vi "golpi_mpc_load_packages.vi"(8 "error in":errorcluster, 11 "golpi session":T1={"GOLPI ref"={"pipe handle"={"lv_proc.dll file path"=path "", "process instance handle"=[], "debug mode"=FALSE, "debug data"=[]}, "fast read timeout [ms]"=500, "fast read settle time [ms]"=10, "fast read to multiple [ms]"=1, "max elements per input line"=100, "slow read timeout [ms]"=5000, "stdin double format specifier"="%_16e", "max elements per stdout output column"=100, "console mode bitstream"=FALSE, "bitstream first read timeout [ms]"=1000, "bitstream read timeout [ms]"=50, "struct transfer possible"=FALSE, "matlab mode"=FALSE}, "idn str"="", "octave path"=path "C:/Octave364/Octave3.6.4_gcc4.6.2/bin", "work path"=path "C:/Octave364/Octave3.6.4_gcc4.6.2/bin", "start timeout [ms]"=15000, "clr cache"=FALSE, "console"=FALSE, "binary"=FALSE, "semaphore"=refnum, "initial command"="", "exit command"="", "matlab"=FALSE, "pkg list"=[]}) -> (0 "error out":errorcluster, 3 "golpi out":T1={"GOLPI ref"={"pipe handle"={"lv_proc.dll file path"=path "", "process instance handle"=[], "debug mode"=FALSE, "debug data"=[]}, "fast read timeout [ms]"=500, "fast read settle time [ms]"=10, "fast read to multiple [ms]"=1, "max elements per input line"=100, "slow read timeout [ms]"=5000, "stdin double format specifier"="%_16e", "max elements per stdout output column"=100, "console mode bitstream"=FALSE, "bitstream first read timeout [ms]"=1000, "bitstream read timeout [ms]"=50, "struct transfer possible"=FALSE, "matlab mode"=FALSE}, "idn str"="", "octave path"=path "C:/Octave364/Octave3.6.4_gcc4.6.2/bin", "work path"=path "C:/Octave364/Octave3.6.4_gcc4.6.2/bin", "start timeout [ms]"=15000, "clr cache"=FALSE, "console"=FALSE, "binary"=FALSE, "semaphore"=refnum, "initial command"="", "exit command"="", "matlab"=FALSE, "pkg list"=[]})   [LabVIEW 2020, in "GOLPI Multi Process.lvlib"]
doc: "Multi-process GOLPI internal function: Tries to load packages listed in GOLPI session."
uses:
  GOLPI Multi Process.lvlib
  golpi_session.ctl
  GOLPI reference Type Def.ctl
  Pipe Handle.ctl
  GOLPI library.lvlib
  LV Process library.lvlib
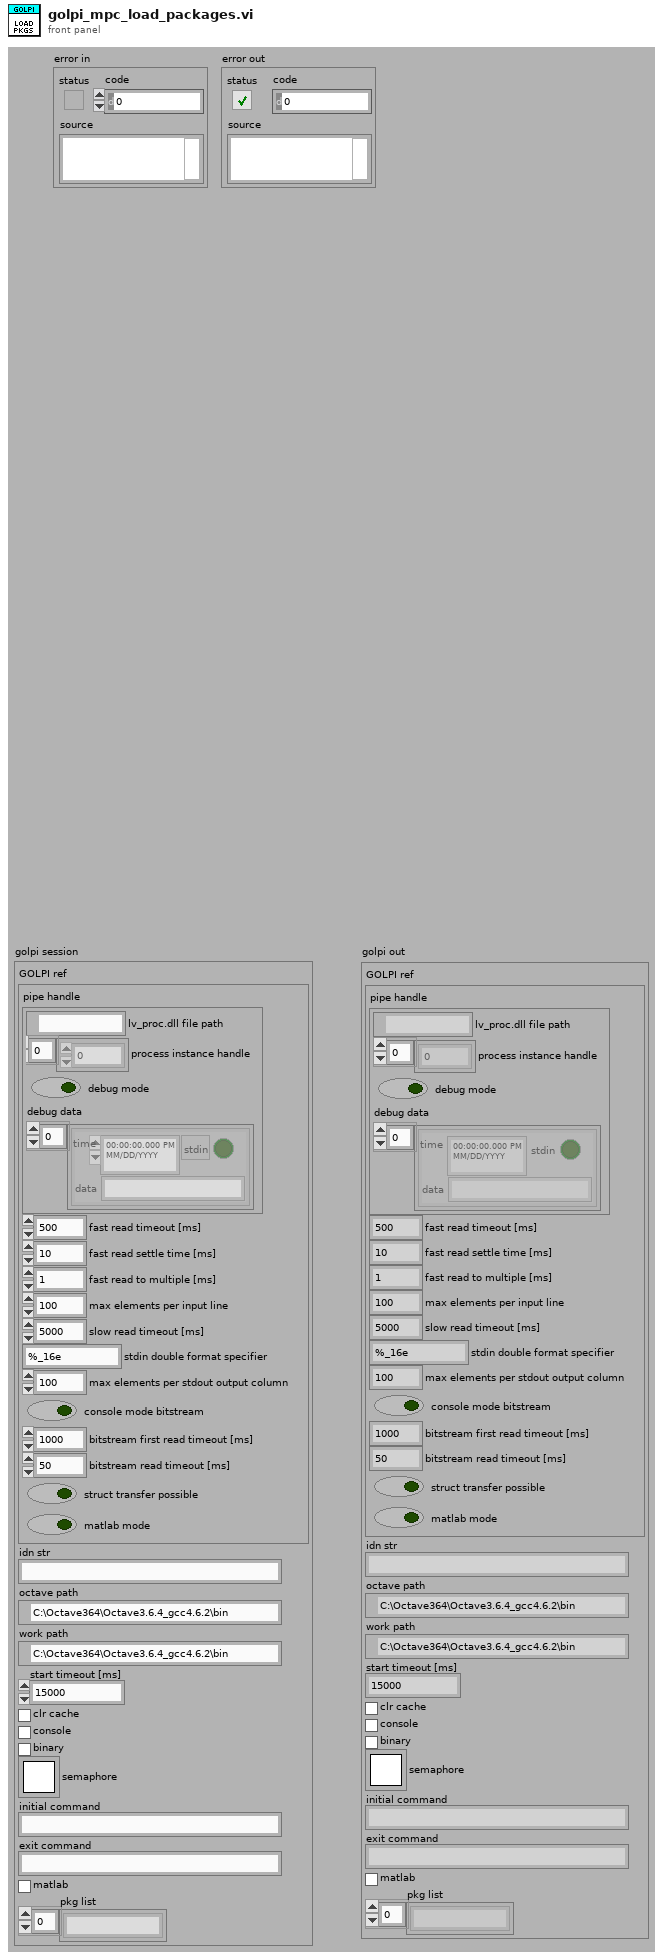
[diagram p1: front panel]
types:
  T1 = typedef "GOLPI Multi Process.lvlib/golpi_session.ctl" = cluster{"GOLPI ref":T2, "idn str":string, "octave path":path, "work path":path, "start timeout [ms]":u32, "clr cache":bool, "console":bool, "binary":bool, "semaphore":T4, "initial command":string, "exit command":string, "matlab":bool, "pkg list":string[]}
  T2 = typedef "GOLPI library.lvlib/GOLPI reference Type Def.ctl" = cluster{"pipe handle":T3, "fast read timeout [ms]":u32, "fast read settle time [ms]":u32, "fast read to multiple [ms]":u32, "max elements per input line":u32, "slow read timeout [ms]":u32, "stdin double format specifier":string, "max elements per stdout output column":u32, "console mode bitstream":bool, "bitstream first read timeout [ms]":u32, "bitstream read timeout [ms]":u32, "struct transfer possible":bool, "matlab mode":bool}
  T3 = typedef "LV Process library.lvlib/Pipe Handle.ctl" = cluster{"lv_proc.dll file path":path, "process instance handle":u32[], "debug mode":bool, "debug data":cluster{"time":timestamp, "stdin":bool, "data":string}[]}
  T4 = typedef "Semaphore RefNum" = refnum<k1>
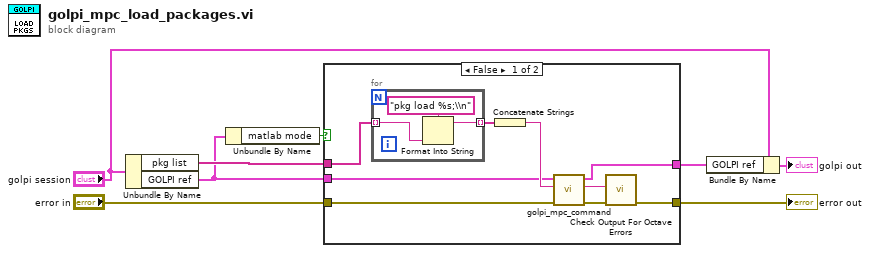
[diagram p0: block diagram]
diagram:
  n1 = Unbundle By Name("golpi session") -> ("pkg list"=w6:string[], "GOLPI ref"=w2:T2)
  n2 = Unbundle By Name(w2) -> ("matlab mode"=w1:bool)
  n3 = case shown="False" w1 {
    tunnel: [w17 w22] -> w8
    tunnel: "error in" -> [w16 w22]
    tunnel: w6 -> [w13 _]
    tunnel: [w10 w21] -> w4
    tunnel: w2 -> [w9 w21]
    frame False {
      n4 = for {
        tunnel: w13 -> [w18] mode=indexing
        tunnel: [w19] -> w12 mode=indexing
        n5 = Format Into String(format string="pkg load %s;\\n", w18) -> (resulting string=w19:string)  [unwired: 2 in, 1 out]
      }
      n6 = Concatenate Strings(w12) -> (w11:string)
      n7 = call "golpi_mpc_command.vi"("error in"=w16, "command"=w11, "GOLPI ref in"=w9) -> ("error out"=w15:errorcluster, "read buffer"=w14:string, "GOLPI ref. out"=w10:T2)  [unwired: 6 in]
      n8 = call "Check Output For Octave Errors.vi"("error in"=w15, "read buffer"=w14) -> ("error out"=w17:errorcluster)  [unwired: 9 in]
    }
    frame True {
    }
  }
  "error out" <- w8
  n9 = Bundle By Name(cluster="golpi session", "GOLPI ref"=w4) -> (→"golpi out":T1)
